vi "Init.vi"(3 "Container State":T7, 4 "Previous State":variant, 5 "Previous Version":T6) -> (2 "Current State":T1={"Nspeakers"=0, "actions"=[], "Wspeaker"=13, "Wmic"=13, "sel mic"=13, "hover"={"type"=enum."None", "index"=0}, "locked"=FALSE, "states"=[], "sel speak"=13, "selected"=refnum, "Events"={"Mic change"=refnum, "Selection change"=refnum}})   [LabVIEW 2015, in "HRTF Config.xctl"]
uses:
  HRTF Config.xctl
  State.vi
  Hover Data.ctl
  Hover Item.ctl
  Speaker State.ctl
  Events.ctl
  Selection changed.ctl
  <vilib>/_xctls/Container State.ctl
  <vilib>/_xctls/Version.ctl
  <vilib>/_xctls/XControlSupport.lvlib
panel:
  in  "Default Indicator State":T1={"Nspeakers"=0, "actions"=[], "Wspeaker"=13, "Wmic"=13, "sel mic"=13, "hover"={"type"=enum."None", "index"=0}, "locked"=FALSE, "states"=[], "sel speak"=13, "selected"=refnum, "Events"={"Mic change"=refnum, "Selection change"=refnum}}
  in  "Default Control State":T1={"Nspeakers"=13, "actions"=[], "Wspeaker"=28, "Wmic"=8, "sel mic"=0, "hover"={"type"=enum."None", "index"=0}, "locked"=FALSE, "states"=[], "sel speak"=13, "selected"=refnum, "Events"={"Mic change"=refnum, "Selection change"=refnum}}
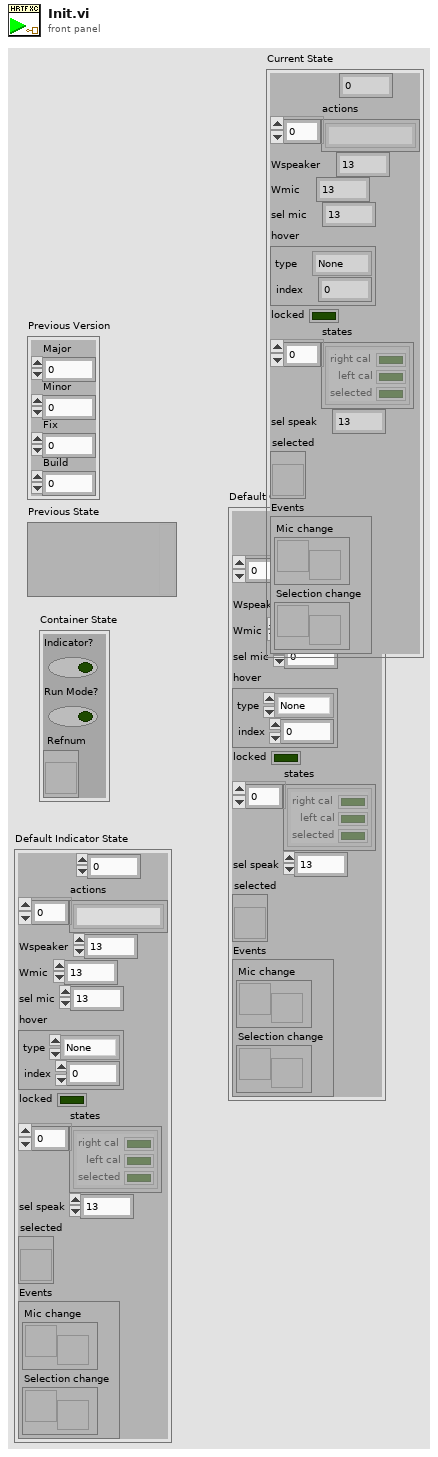
[diagram p1: front panel]
types:
  T1 = typedef "HRTF Config.xctl/State.vi" = cluster{"Nspeakers":i32, "actions":string[], "Wspeaker":i32, "Wmic":i32, "sel mic":i32, "hover":T2, "locked":bool, "states":T4[], "sel speak":i32, "selected":refnum<vi>, "Events":T5}
  T2 = typedef "HRTF Config.xctl/Hover Data.ctl" = cluster{"type":T3, "index":i32}
  T3 = typedef "HRTF Config.xctl/Hover Item.ctl" = enum16{"None", "Speaker", "Mic"}
  T4 = typedef "HRTF Config.xctl/Speaker State.ctl" = cluster{"right cal":bool, "left cal":bool, "selected":bool}
  T5 = typedef "HRTF Config.xctl/Events.ctl" = cluster{"Mic change":refnum<user-event>, "Selection change":refnum<user-event>}
  T6 = typedef "XControlSupport.lvlib/Version.ctl" = cluster{"Major":u16, "Minor":u16, "Fix":u16, "Build":u16}
  T7 = typedef "XControlSupport.lvlib/Container State.ctl" = cluster{"Indicator?":bool, "Run Mode?":bool, " Refnum":refnum<vi>}
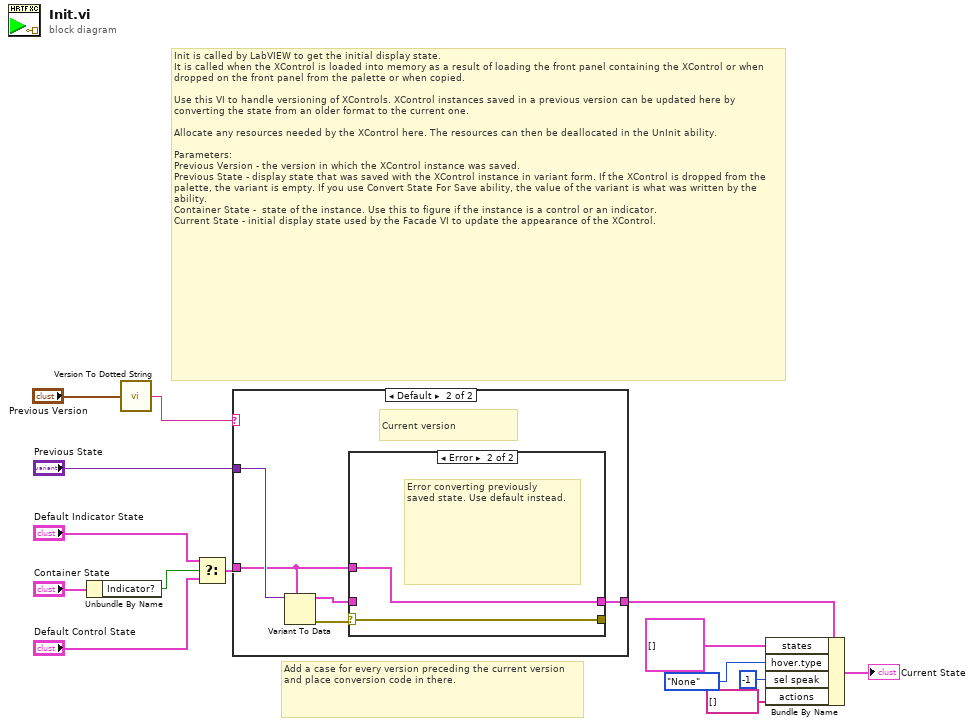
[diagram p0: block diagram]
diagram:
  # "Add a case for every version preceding the current version and place conversion code in there."
  # "Init is called by LabVIEW to get the initial display state.\nIt is called when the XControl is loaded into memory as a result of loading the front panel containing the XControl or when dropped on the front panel from the palette or when copied.\n\nUse this VI to handle versioning of XControls. XControl instances saved in a previous version can be updated here by converting the state from an older format to the current one.\n\nAllocate any resources needed by the XControl here. The resources can then be deallocated in the UnInit ability.\n\nParameters:\nPrevious Version - the version in which the XControl instance was saved.\nPrevious State - display state that was saved with the XControl instance in variant form. If the XControl is dropped from the palette, the variant is empty. If you use Convert State For Save ability, the value of the variant is what was written by the ability. \nContainer State -  state of the instance. Use this to figure if the instance is a control or an indicator.\nCurrent State - initial display state used by the Facade VI to update the appearance of the XControl."
  n1 = Unbundle By Name("Container State") -> ("Indicator?"=w9:bool)
  n2 = call <vilib>:"Version To Dotted String.vi"("Version"="Previous Version") -> ("String Version"=w6:string)
  n3 = Select(t="Default Indicator State", s=w9, f="Default Control State") -> (s? t:f=w8:T1)
  n4 = case shown="Default" w6 {
    tunnel: "Previous State" -> [_ w20]
    tunnel: [w15 w16] -> w13
    tunnel: w8 -> [w15 w17]
    frame "0.0.0.0" {
      # "Just created, use default state"
    }
    frame Default {
      # "Current version"
      n5 = Variant To Data(type=w17, Variant=w20) -> (data=w18:T1, error out=w19:errorcluster)  [unwired: 1 in]
      n6 = case shown="Error" w19 {
        selector: w19 -> [w22 w23]
        tunnel: w18 -> [w21 _]
        tunnel: [w21 w24] -> w16
        tunnel: w17 -> [_ w24]
        tunnel: [w22 w23] -> _
        frame No Error {
        }
        frame Error {
          # "Error converting previously \nsaved state. Use default instead."
        }
      }
    }
  }
  n7 = Bundle By Name(cluster=w13, "states"=T4[] [], "hover.type"=Hover_Item."None", "sel speak"=-1, "actions"=string[] []) -> (→"Current State":T1)
